vi "PP.vi"() -> ()   [LabVIEW 2018]
uses:
  <vilib>/LabVIEW Interface for Arduino/Type Defs/Pin Mode.ctl
  <vilib>/LabVIEW Interface for Arduino/Type Defs/Connection Type.ctl
  <vilib>/LabVIEW Interface for Arduino/Type Defs/Board Type.ctl
  <vilib>/LabVIEW Interface for Arduino/LabVIEW Interface for Arduino.lvlib
panel:
  in  "ROJO":dbl
  out "Servo 0":dbl(knob) scale=0.0..90.0
  in  "VERDE":dbl
  out "Rojo":bool
  out "Verde":bool
  in  "Detener":bool
  # "Proyecto Final: Estacionamiento"
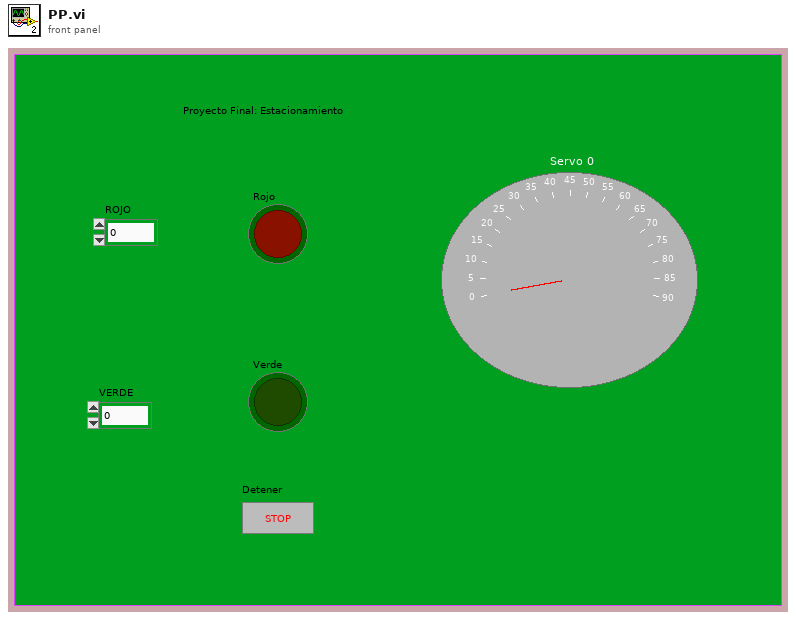
[diagram p1: front panel]
types:
  T1 = typedef "LabVIEW Interface for Arduino.lvlib/Board Type.ctl" = enum16{"Uno", "Dimuelanove w/Atmega 328", "Mega 2560"}
  T2 = typedef "LabVIEW Interface for Arduino.lvlib/Connection Type.ctl" = enum8{"USB / Serial", "XBEE", "BlueSmirf (Bluetooth)"}
  T3 = typedef "LabVIEW Interface for Arduino.lvlib/Pin Mode.ctl" = enum8{"Input", "Output"}
  T4 = typedef "LabVIEW Interface for Arduino.lvlib/Arduino Resource.ctl" = cluster{"VISA resource":refnum<visa-resource-name>, "Board Type":T1, "Connection Type":enum8{"USB / Serial"}, "Bytes Per Packet (15)":u8}
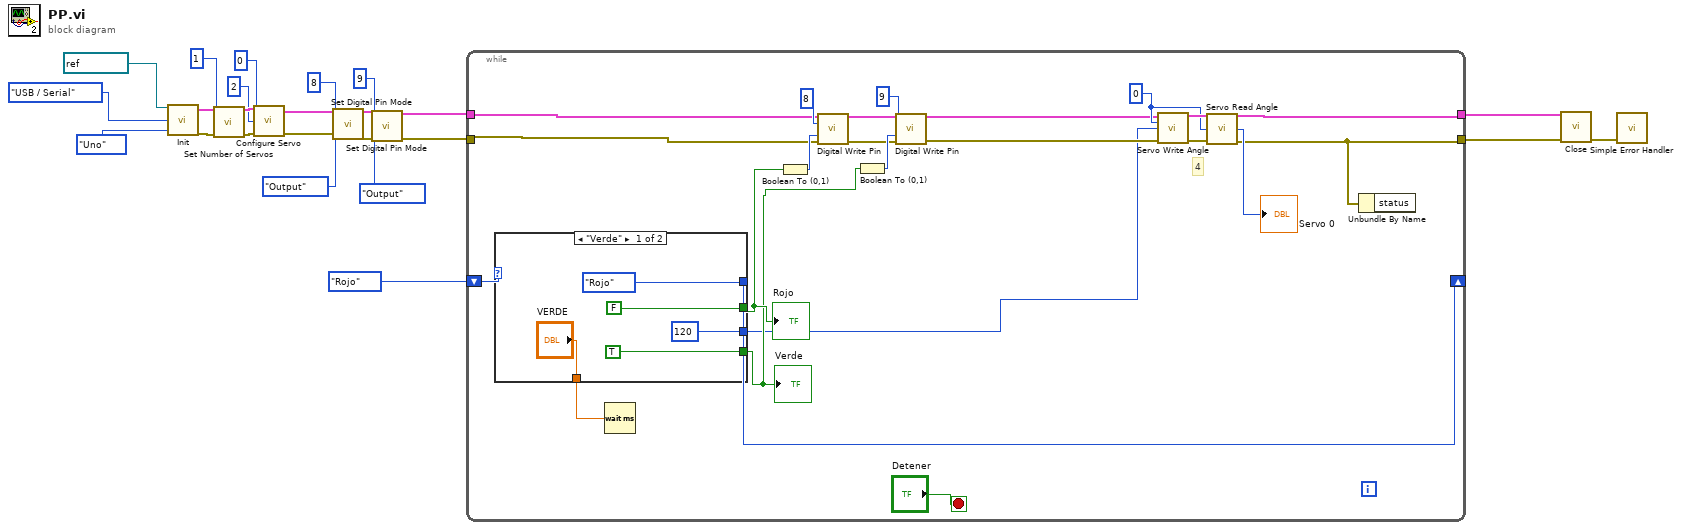
[diagram p0: block diagram]
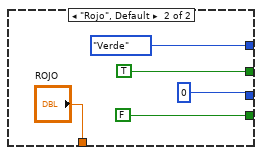
[diagram p2: hidden frame]
diagram:
  n1 = call <vilib>:"Init.vi"("VISA resource"=refnum<visa-resource-name> "COM9", "Board Type (Uno)"=Board_Type."Uno", "Connection Type (USB/Serial)"=Connection_Type."USB / Serial") -> ("Arduino Resource"=w9:T4, "error out"=w8:errorcluster)  [unwired: 15 in]
  n2 = call <vilib>:"Set Number of Servos.vi"("Arduino Resource"=w9, "Number Of Servos (1)"=u8 1, "error in"=w8) -> ("Arduino Resource"=w14:T4, "error out"=w13:errorcluster)  [unwired: 11 in]
  n3 = call <vilib>:"Configure Servo.vi"("Arduino Resource"=w14, "Servo Number (0)"=u8 0, "DIO Pin (2)"=u8 2, "error in"=w13) -> ("Arduino Resource"=w11:T4, "error out"=w10:errorcluster)  [unwired: 10 in]
  n4 = call <vilib>:"Set Digital Pin Mode.vi"("Arduino Resource"=w11, "Digital I/O Pin"=u8 8, "Pin Mode (Input)"=Pin_Mode."Output", "error in"=w10) -> ("Arduino Resource"=w4:T4, "error out"=w3:errorcluster)  [unwired: 10 in]
  n5 = call <vilib>:"Set Digital Pin Mode.vi"("Arduino Resource"=w4, "Digital I/O Pin"=u8 9, "Pin Mode (Input)"=Pin_Mode."Output", "error in"=w3) -> ("Arduino Resource"=w2:T4, "error out"=w1:errorcluster)  [unwired: 10 in]
  n6 = while {
    shift-right: [w45] -> _
    shift-left: enum16{"Rojo", "Amarillo", "Verde"}."Rojo" -> [w46]
    tunnel: w2 -> [w26]
    tunnel: w1 -> [w25]
    tunnel: [w29] -> w20
    tunnel: [w28] -> w19
    stop <- "Detener" stop-if-true
    w33 = u8 0 ("Servo Number")
    # "4"
    n7 = case shown="\"Verde\"" w46 {
      tunnel: [enum16{"Rojo", "Amarillo", "Verde"}."Rojo" enum16{"Rojo", "Amarillo", "Verde"}."Verde"] -> w45
      tunnel: [FALSE TRUE] -> w39
      tunnel: [TRUE FALSE] -> w38
      tunnel: ["VERDE" "ROJO"] -> w44
      tunnel: [u8 120 ("Angle (Degrees)") u8 0 ("Angle (Degrees)")] -> w27
      frame "Verde" {
      }
      frame "Rojo", Default {
      }
    }
    "Rojo" <- w39
    "Verde" <- w38
    n8 = Wait (ms) ("Wait (s)")(milliseconds to wait=w44) -> ()  [unwired: 1 out]
    n9 = Boolean To (0,1)(Boolean=w39) -> (0, 1=w41:i16)
    n10 = call <vilib>:"Digital Write Pin.vi"("Arduino Resource"=w26, "Digital I/O Pin (0)"=u8 8, "Value (0)"=w41, "error in"=w25) -> ("Arduino Resource"=w37:T4, "error out"=w36:errorcluster)  [unwired: 10 in]
    n11 = Boolean To (0,1)(Boolean=w38) -> (0, 1=w40:i16)
    n12 = call <vilib>:"Digital Write Pin.vi"("Arduino Resource"=w37, "Digital I/O Pin (0)"=u8 9, "Value (0)"=w40, "error in"=w36) -> ("Arduino Resource"=w31:T4, "error out"=w30:errorcluster)  [unwired: 10 in]
    n13 = call <vilib>:"Servo Write Angle.vi"("Arduino Resource"=w31, "Servo Number"=w33, "Angle (Degrees)"=w27, "error in"=w30) -> ("Arduino Resource"=w35:T4, "error out"=w34:errorcluster)  [unwired: 10 in]
    n14 = call <vilib>:"Servo Read Angle.vi"("Arduino Resource"=w35, "Servo Number"=w33, "error in"=w34) -> ("Arduino Resource"=w29:T4, "Angle (Degrees)"=→"Servo 0":u8, "error out"=w28:errorcluster)  [unwired: 10 in]
    n15 = Unbundle By Name(w28) -> ()  [unwired: 1 out]
  }
  n16 = call <vilib>:"Close.vi"("Arduino Resource"=w20, "error in"=w19) -> ("error out"=w18:errorcluster)  [unwired: 13 in]
  n17 = call <vilib>:"Simple Error Handler.vi"("error in (no error)"=w18) -> ()  [unwired: 4 in, 5 out]
